vi "VisionRobotWrapper.vi"(2 "error in (no error)":errorcluster) -> ()   [LabVIEW 2012]
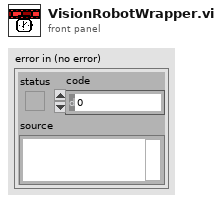
[diagram p1: front panel]
types:
  T1 = typedef "Image Type" = u32
  T2 = typedef "WPI_CameraDevRef.ctl" = cluster{"Camera Address":string, "CameraStatus":errorcluster, "Acquire Image Notifier":refnum<notifier>}
  T3 = typedef "IMAQ Image.ctl" = refnum<image>
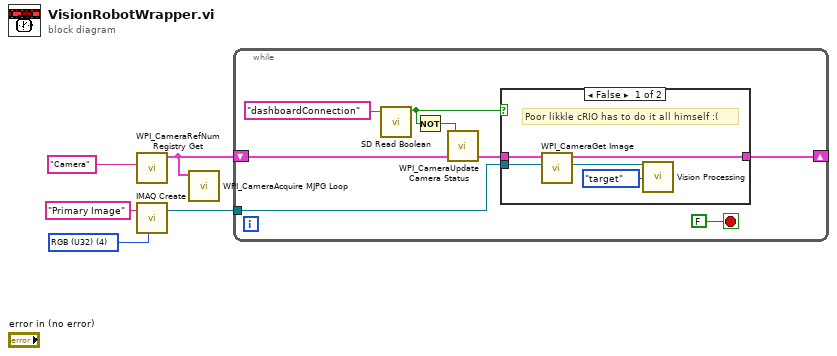
[diagram p0: block diagram]
diagram:
  w3 = T1 4 items=["Grayscale (U8)", "Grayscale (I16)", "Grayscale (SGL)", "Complex (CSG)", "RGB (U32)", "HSL (U32)", "RGB (U64)"] ("Image Type")
  n1 = call <vilib>:"WPI_CameraRefNum Registry Get.vi"("refnum name"="Camera") -> ("CameraDevRef"=w1:T2)  [unwired: 1 in, 9 out]
  n2 = call "IMAQ Create"("Image Name"="Primary Image", "Image Type"=w3) -> ("New Image"=w2:T3)  [unwired: 2 in, 2 out]
  n3 = call <vilib>:"WPI_CameraAcquire MJPG Loop.vi"("CameraDevRef"=w1) -> ()  [unwired: 11 in]
  n4 = while {
    tunnel: w2 -> [w8]
    shift-right: [w6] -> _
    shift-left: w1 -> [w12]
    stop <- FALSE stop-if-true
    n5 = call <vilib>:"SD Read Boolean.vi"("Name"="dashboardConnection") -> ("Boolean"=w10:bool)  [unwired: 8 in, 2 out]
    n6 = Not(x=w10) -> (.not. x?=w11:bool)
    n7 = call <vilib>:"WPI_CameraUpdate Camera Status.vi"("CameraDevRef In"=w12, "Enable Vision"=w11) -> ("CameraDevRef Out"=w9:T2)  [unwired: 3 in]
    n8 = case shown="False" w10 {
      tunnel: w9 -> [w17 w19]
      tunnel: w8 -> [w16 _]
      tunnel: [w14 w19] -> w6
      frame False {
        # "Poor likkle cRIO has to do it all himself :("
        n9 = call <vilib>:"WPI_CameraGet Image.vi"("Image"=w16, "CameraDevRef"=w17) -> ("Image Out"=w15:T3, "CameraDevRef Out"=w14:T2)  [unwired: 1 in, 7 out]
        n10 = call "Vision Processing.vi"("New Image"=w15, "Enum"=enum16{"target", "disc"}."target") -> ()  [unwired: 13 in, 1 out]
      }
      frame True {
        # "Oh, you big sexy\nfast Lenovo... you go girl!"
      }
    }
  }
